vi "rcpacini_v_representation.vi"(6 "Variant in":variant, 7 "Shift Pressed?":bool, 8 "error in (no error)":errorcluster, 10 "QD Combo Box Ref":refnum<vi>, 11 "QD Launch VI Ref":refnum<vi>) -> (0 "error out":errorcluster, 4 "Variant out":variant)   [LabVIEW 2019]
doc: "Change the selected numeric or string control/constant representation, radix and modifiers using the quick drop text formatted as : \n<b>TYPE[ MODS...]</b>\n<b>TYPE</b> = 'u8', 'u16', 'u32', 'u64', 'i8', 'i16', 'i32', 'i64', 'sgl', 'dbl', 'ext'\n<b>MODS</b> = 'x':hex, 'd':dec/default, 'b':bin/backslash, 'h':hide inc/dec buttons \n\n<b>Examples:</b>\nNumeric selected + <b>\"u8 h x\"</b> = Unsigned 8-bit representation, display radix as hex and inc/dec buttons hidden\nString selected + <b>\"b\"</b> = Show display radix in backslash\n\nDefault Shortcut - [V]"
uses:
  <vilib>/numeric/LVNumericRepresentation.ctl
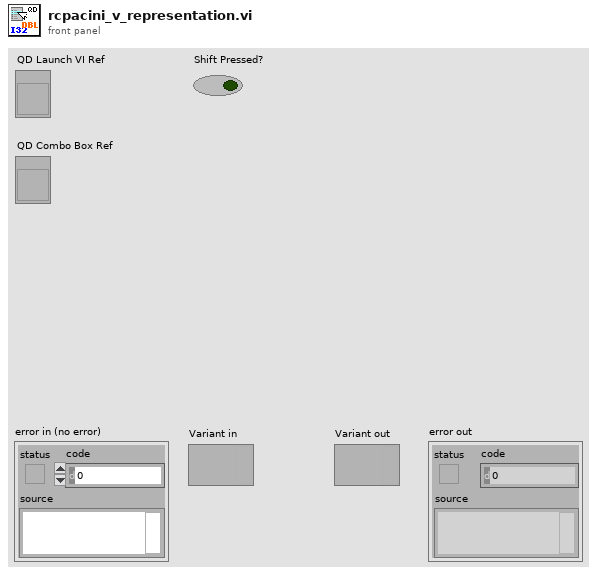
[diagram p1: front panel]
types:
  T1 = typedef "LVNumericRepresentation.ctl" = enum32{"Extended Precision", "Double Precision", "Single Precision", "Long", "Word", "Byte", "Unsigned Long", "Unsigned Word", "Unsigned Byte", "Complex Extended", "Complex Double", "Complex Single", "Quad", "Unsigned Quad", "Fixed-Point"}
  T2 = enum8{"none", "toggle", "decimal", "hex", "binary"}
  T3 = cluster{"DigitalCst":refnum<vi>[], "EnumCst":refnum<vi>[], "RingCst":refnum<vi>[], "StringCst":refnum<vi>[], "Digitals":refnum<vi>[], "Enums":refnum<vi>[], "Rings":refnum<vi>[], "Strings":refnum<vi>[]}
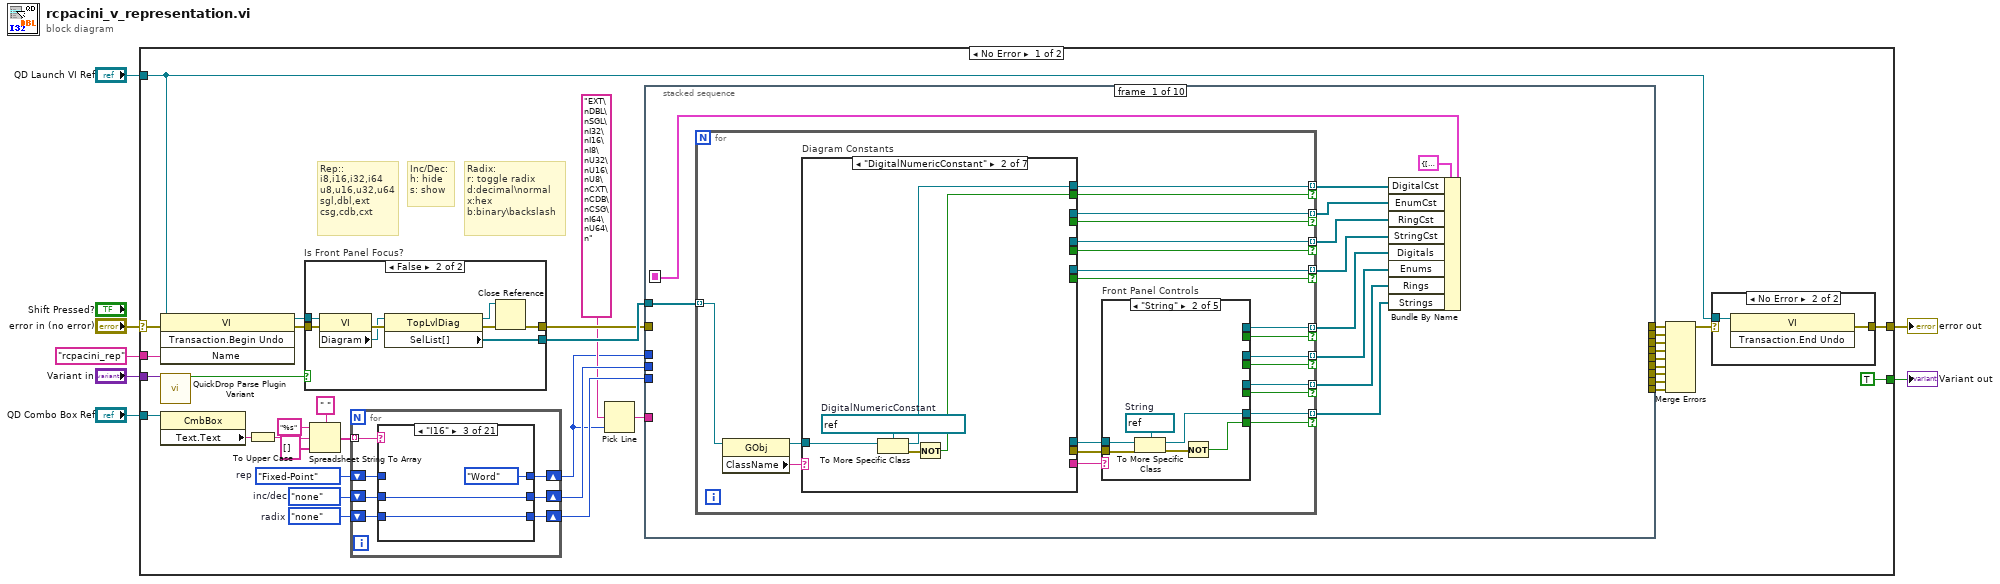
[diagram p0: block diagram]
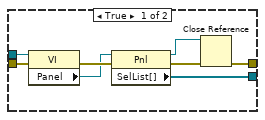
[diagram p2: hidden frame]
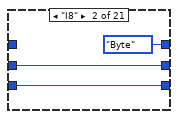
[diagram p4: hidden frame]
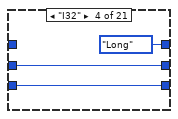
[diagram p5: hidden frame]
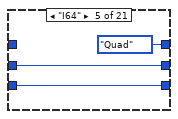
[diagram p6: hidden frame]
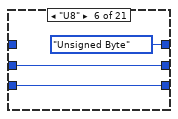
[diagram p7: hidden frame]
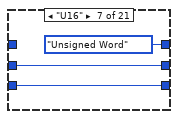
[diagram p8: hidden frame]
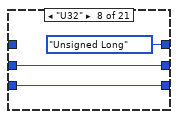
[diagram p9: hidden frame]
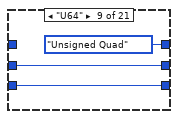
[diagram p10: hidden frame]
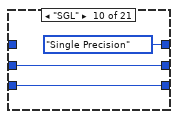
[diagram p11: hidden frame]
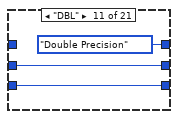
[diagram p12: hidden frame]
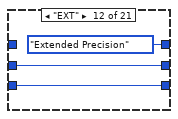
[diagram p13: hidden frame]
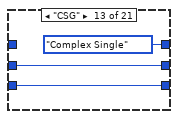
[diagram p14: hidden frame]
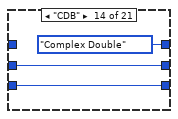
[diagram p15: hidden frame]
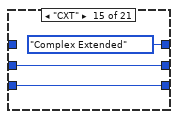
[diagram p16: hidden frame]
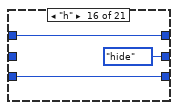
[diagram p17: hidden frame]
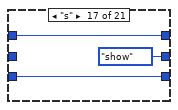
[diagram p18: hidden frame]
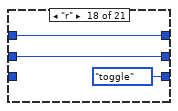
[diagram p19: hidden frame]
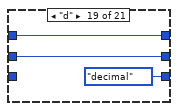
[diagram p20: hidden frame]
diagram:
  n1 = case shown="No Error" "error in (no error)" {
    selector: "error in (no error)" -> [w43 w621]
    tunnel: [w42 w621] -> w1
    tunnel: "QD Launch VI Ref" -> [w36 _]
    tunnel: "rcpacini_rep" ("Undo Name") -> [w41 _]
    tunnel: "Variant in" -> [w9 _]
    tunnel: "QD Combo Box Ref" -> [w37 _]
    tunnel: [TRUE _] -> w2
    frame No Error {
      w26 = enum8{"none", "show", "hide"}."none"  # inc/dec
      w27 = T2."none"  # radix
      w28 = LVNumericRepresentation."Fixed-Point"  # rep
      # "Radix:\nr: toggle radix\nd:decimal\\normal\nx:hex\nb:binary\\backslash"
      # "Inc/Dec:\nh: hide\ns: show"
      # "Rep::\ni8,i16,i32,i64\nu8,u16,u32,u64\nsgl,dbl,ext\ncsg,cdb,cxt"
      n2 = invoke class="VI" method="Transaction.Begin Undo"(reference=w36, error in=w43, "Name"=w41) -> (reference out=w39:refnum<vi>, error out=w40:errorcluster)  [unwired: 1 in, 2 out]
      n3 = call <vilib>:"QuickDrop Parse Plugin Variant.vi"("QDKS Variant in"=w9) -> ("QD Launch VI Panel?"=w8:bool)  [unwired: 12 in, 2 out]
      n4 = property class="CmbBox"(reference=w37) -> ("Text.Text"=w35:string)  [unwired: 1 in, 2 out]
      n5 = To Upper Case(1:w35) -> (0:w34:string)
      n6 = case "Is Front Panel Focus?" shown="False" w8 {
        tunnel: w40 -> [w51 w59]
        tunnel: w39 -> [w50 w58]
        tunnel: [w45 w53] -> w25
        tunnel: [w44 w52] -> w30
        frame True {
          n7 = property class="VI"(reference=w50, error in=w51) -> (error out=w49:errorcluster, "Panel"=w48:refnum<vi>)  [unwired: 1 out]
          n8 = property class="Pnl"(reference=w48, error in=w49) -> (reference out=w46:refnum<vi>, error out=w47:errorcluster, "SelList[]"=w44:refnum<vi>[])
          n9 = Close Reference(reference=w46, error in (no error)=w47) -> (error out=w45:errorcluster)
        }
        frame False {
          n10 = property class="VI"(reference=w58, error in=w59) -> (error out=w57:errorcluster, "Diagram"=w56:refnum<vi>)  [unwired: 1 out]
          n11 = property class="TopLvlDiag"(reference=w56, error in=w57) -> (reference out=w54:refnum<vi>, error out=w55:errorcluster, "SelList[]"=w52:refnum<vi>[])
          n12 = Close Reference(reference=w54, error in (no error)=w55) -> (error out=w53:errorcluster)
        }
      }
      n13 = Spreadsheet String To Array(delimiter (Tab)=" ", format string="%s", spreadsheet string=w34, array type (2D Dbl)=string[] []) -> (array=w29:string[])
      n14 = for {
        tunnel: w29 -> [w66] mode=indexing
        shift-right: [w64] -> w11
        shift-left: w28 -> [w65]
        shift-right: [w63] -> w23
        shift-left: w26 -> [w62]
        shift-right: [w60] -> w22
        shift-left: w27 -> [w61]
        n15 = case shown="\"I16\"" w66 {
          tunnel: w65 -> [w69 _ _ _ _ _ _ _ _ _ _ _ _ _ _ w114 w117 w120 w123 w126 w129]
          tunnel: [w69 LVNumericRepresentation."Byte" ("Representation") LVNumericRepresentation."Word" ("Representation") LVNumericRepresentation."Long" ("Representation") LVNumericRepresentation."Quad" ("Representation") LVNumericRepresentation."Unsigned Byte" ("Representation") LVNumericRepresentation."Unsigned Word" ("Representation") LVNumericRepresentation."Unsigned Long" ("Representation") LVNumericRepresentation."Unsigned Quad" ("Representation") LVNumericRepresentation."Single Precision" ("Representation") LVNumericRepresentation."Double Precision" ("Representation") LVNumericRepresentation."Extended Precision" ("Representation") LVNumericRepresentation."Complex Single" ("Representation") LVNumericRepresentation."Complex Double" ("Representation") LVNumericRepresentation."Complex Extended" ("Representation") w114 w117 w120 w123 w126 w129] -> w64
          tunnel: [w68 w71 w74 w77 w80 w83 w86 w89 w92 w95 w98 w101 w104 w107 w110 enum8{"none", "show", "hide"}."hide" ("inc/dec") enum8{"none", "show", "hide"}."show" ("inc/dec") w119 w122 w125 w128] -> w63
          tunnel: w62 -> [w68 w71 w74 w77 w80 w83 w86 w89 w92 w95 w98 w101 w104 w107 w110 _ _ w119 w122 w125 w128]
          tunnel: [w67 w70 w73 w76 w79 w82 w85 w88 w91 w94 w97 w100 w103 w106 w109 w113 w116 T2."toggle" ("radix") T2."decimal" ("radix") T2."hex" ("radix") T2."binary" ("radix")] -> w60
          tunnel: w61 -> [w67 w70 w73 w76 w79 w82 w85 w88 w91 w94 w97 w100 w103 w106 w109 w113 w116 _ _ _ _]
          frame Default {
          }
          frame "I8" {
          }
          frame "I16" {
          }
          frame "I32" {
          }
          frame "I64" {
          }
          frame "U8" {
          }
          frame "U16" {
          }
          frame "U32" {
          }
          frame "U64" {
          }
          frame "SGL" {
          }
          frame "DBL" {
          }
          frame "EXT" {
          }
          frame "CSG" {
          }
          frame "CDB" {
          }
          frame "CXT" {
          }
          frame "h" {
          }
          frame "s" {
          }
          frame "r" {
          }
          frame "d" {
          }
          frame "x" {
          }
          frame "b" {
          }
        }
      }
      n16 = Pick Line(multi-line string="EXT\nDBL\nSGL\nI32\nI16\nI8\nU32\nU16\nU8\nCXT\nCDB\nCSG\nI64\nU64\n", line index=w11) -> (output string=w10:string)  [unwired: 1 in]
      n17 = stacked-sequence {
        seq-local: [w130 _ _ _ _ _ _ _ _ _] -> [_ w220 w304 w334 w364 w414 w501 w532 w566 _]
        tunnel: w30 -> [w140 _ _ _ _ _ _ _ _ w616]
        tunnel: w25 -> [_ w219 w303 w333 w363 w413 w500 w531 w565 w615]
        tunnel: w11 -> [_ w224 w306 w336 _ w417 w503 w534 _ _]
        tunnel: w23 -> [_ w223 _ _ w365 w416 w502 w533 w567 _]
        tunnel: w22 -> [_ w222 _ _ w366 w415 _ _ w568 _]
        tunnel: [_ w218 _ _ _ _ _ _ _ _] -> w24
        tunnel: w10 -> [_ w221 w305 w335 _ _ _ _ _ _]
        tunnel: [_ _ w302 _ _ _ _ _ _ _] -> w21
        tunnel: [_ _ _ w332 _ _ _ _ _ _] -> w20
        tunnel: [_ _ _ _ w362 _ _ _ _ _] -> w19
        tunnel: [_ _ _ _ _ w412 _ _ _ _] -> w18
        tunnel: [_ _ _ _ _ _ w499 _ _ _] -> w17
        tunnel: [_ _ _ _ _ _ _ w530 _ _] -> w16
        tunnel: [_ _ _ _ _ _ _ _ w564 _] -> w15
        tunnel: [_ _ _ _ _ _ _ _ _ w614] -> w14
        frame #0 {
          n18 = for {
            tunnel: w140 -> [w162] mode=indexing
            tunnel: [w159] -> w139 mode=indexing if=w158
            tunnel: [w157] -> w138 mode=indexing if=w156
            tunnel: [w155] -> w137 mode=indexing if=w154
            tunnel: [w153] -> w136 mode=indexing if=w152
            tunnel: [w148] -> w132 mode=indexing if=w147
            tunnel: [w146] -> w135 mode=indexing if=w145
            tunnel: [w144] -> w134 mode=indexing if=w143
            tunnel: [w142] -> w133 mode=indexing if=w141
            n19 = property class="GObj"(reference=w162) -> (reference out=w160:refnum<vi>, "ClassName"=w161:string)  [unwired: 1 in, 1 out]
            n20 = case "Diagram Constants" shown="\"DigitalNumericConstant\"" w161 {
              selector: w161 -> [_ _ _ _ _ _ w216]
              tunnel: w160 -> [_ w190 w195 w200 w205 w214 w217]
              tunnel: [_ w189 _ _ _ _ _] -> w159
              tunnel: [_ w187 _ _ _ _ _] -> w158
              tunnel: [_ _ w193 _ _ _ _] -> w157
              tunnel: [_ _ w192 _ _ _ _] -> w156
              tunnel: [_ _ _ w198 _ _ _] -> w155
              tunnel: [_ _ _ w197 _ _ _] -> w154
              tunnel: [_ _ _ _ w203 _ _] -> w153
              tunnel: [_ _ _ _ w202 _ _] -> w152
              tunnel: [_ _ _ _ _ w209 w216] -> w149
              tunnel: [_ _ _ _ _ w208 w217] -> w151
              tunnel: [_ _ _ _ _ w207 _] -> w150
              frame Default {
              }
              frame "DigitalNumericConstant" {
                w191 = refnum<vi> refnum  # DigitalNumericConstant
                n21 = To More Specific Class(target class=w191, reference=w190) -> (specific class reference=w189:refnum<vi>, error out=w188:errorcluster)  [unwired: 1 in]
                n22 = Not(x=w188) -> (.not. x?=w187:bool)
              }
              frame "EnumConstant" {
                w196 = refnum<vi> refnum  # EnumConstant
                n23 = To More Specific Class(target class=w196, reference=w195) -> (specific class reference=w193:refnum<vi>, error out=w194:errorcluster)  [unwired: 1 in]
                n24 = Not(x=w194) -> (.not. x?=w192:bool)
              }
              frame "RingConstant" {
                w201 = refnum<vi> refnum  # RingConstant
                n25 = To More Specific Class(target class=w201, reference=w200) -> (specific class reference=w198:refnum<vi>, error out=w199:errorcluster)  [unwired: 1 in]
                n26 = Not(x=w199) -> (.not. x?=w197:bool)
              }
              frame "StringConstant" {
                w206 = refnum<vi> refnum  # StringConstant
                n27 = To More Specific Class(target class=w206, reference=w205) -> (specific class reference=w203:refnum<vi>, error out=w204:errorcluster)  [unwired: 1 in]
                n28 = Not(x=w204) -> (.not. x?=w202:bool)
              }
              frame "ControlTerminal" {
                w215 = refnum<vi> refnum  # ControlTerminal
                n29 = To More Specific Class(target class=w215, reference=w214) -> (specific class reference=w211:refnum<vi>, error out=w213:errorcluster)  [unwired: 1 in]
                n30 = property class="CtrlTerm"(reference=w211, error in=w213) -> (error out=w212:errorcluster, "Control"=w210:refnum<vi>)  [unwired: 1 out]
                n31 = property class="Ctl"(reference=w210, error in=w212) -> (reference out=w208:refnum<vi>, error out=w207:errorcluster, "ClassName"=w209:string)
              }
              frame "Digital", "Enum", "Ring", "String" {
              }
            }
            n32 = case "Front Panel Controls" shown="\"String\"" w149 {
              tunnel: w151 -> [_ w167 w173 w179 w185]
              tunnel: w150 -> [_ w166 w172 w178 w184]
              tunnel: [_ w164 _ _ _] -> w148
              tunnel: [_ w163 _ _ _] -> w147
              tunnel: [_ _ w170 _ _] -> w146
              tunnel: [_ _ w169 _ _] -> w145
              tunnel: [_ _ _ w176 _] -> w144
              tunnel: [_ _ _ w175 _] -> w143
              tunnel: [_ _ _ _ w182] -> w142
              tunnel: [_ _ _ _ w181] -> w141
              frame Default {
              }
              frame "String" {
                w168 = refnum<vi> refnum  # String
                n33 = To More Specific Class(target class=w168, reference=w167, error in=w166) -> (specific class reference=w164:refnum<vi>, error out=w165:errorcluster)
                n34 = Not(x=w165) -> (.not. x?=w163:bool)
              }
              frame "Digital" {
                w174 = refnum<vi> refnum  # Digital
                n35 = To More Specific Class(target class=w174, reference=w173, error in=w172) -> (specific class reference=w170:refnum<vi>, error out=w171:errorcluster)
                n36 = Not(x=w171) -> (.not. x?=w169:bool)
              }
              frame "Enum" {
                w180 = refnum<vi> refnum  # Enum
                n37 = To More Specific Class(target class=w180, reference=w179, error in=w178) -> (specific class reference=w176:refnum<vi>, error out=w177:errorcluster)
                n38 = Not(x=w177) -> (.not. x?=w175:bool)
              }
              frame "Ring" {
                w186 = refnum<vi> refnum  # Ring
                n39 = To More Specific Class(target class=w186, reference=w185, error in=w184) -> (specific class reference=w182:refnum<vi>, error out=w183:errorcluster)
                n40 = Not(x=w183) -> (.not. x?=w181:bool)
              }
            }
          }
          n41 = Bundle By Name(cluster=T3 {"DigitalCst"=[], "EnumCst"=[], "RingCst"=[], "StringCst"=[], "Digitals"=[], "Enums"=[], "Rings"=[], "Strings"=[]} ("refnums"), "DigitalCst"=w139, "EnumCst"=w138, "RingCst"=w137, "StringCst"=w136, "Digitals"=w135, "Enums"=w134, "Rings"=w133, "Strings"=w132) -> (w130:T3)
        }
        frame #1 {
          n42 = Unbundle By Name(w220) -> ("DigitalCst"=w225:refnum<vi>[])
          n43 = for {
            tunnel: w225 -> [w237] mode=indexing
            tunnel: w224 -> [w235]
            tunnel: w223 -> [_]
            tunnel: w222 -> [w234]
            tunnel: w219 -> [w236]
            tunnel: w221 -> [w230]
            shift-right: [w227] -> w218
            shift-left: w219 -> [w226]
            n44 = case shown="Default" w235 {
              selector: w235 -> [_ w298]
              tunnel: w237 -> [w295 w301]
              tunnel: w236 -> [w296 w300]
              tunnel: [w296 w299] -> w229
              tunnel: [w295 w297] -> w228
              frame "Fixed-Point" {
              }
              frame Default {
                n45 = property class="DigCnst"(reference=w301, error in=w300, "Representation"=w298) -> (reference out=w297:refnum<vi>, error out=w299:errorcluster)
              }
            }
            n46 = case shown="\"binary\"" w234 {
              tunnel: w229 -> [w247 w253 w264 w278 w294]
              tunnel: w228 -> [w246 w251 w262 w276 w293]
              tunnel: [w247 w255 w266 w280 w289] -> w233
              tunnel: [w246 w254 w265 w279 w287] -> w231
              frame "none" {
              }
              frame "decimal" {
                n47 = property class="DigCnst"(reference=w251, error in=w253) -> (reference out=w250:refnum<vi>, error out=w252:errorcluster, "Representation"=w249:T1)
                n48 = case shown="\"Long\"..\"Unsigned Byte\", \"Quad\", \"Unsigned Quad\"" w249 {
                  tunnel: [_ "%d" "%#_13g"] -> w248
                  frame "Fixed-Point" {
                  }
                  frame "Long".."Unsigned Byte", "Quad", "Unsigned Quad" {
                  }
                  frame "Extended Precision".."Single Precision", "Complex Extended".."Complex Single" {
                  }
                }
                n49 = property class="DigCnst"(reference=w250, error in=w252, "RadixVis"=TRUE ("Radix Visible?"), "FormatString"=w248) -> (reference out=w254:refnum<vi>, error out=w255:errorcluster)
              }
              frame "hex" {
                n50 = property class="DigCnst"(reference=w262, error in=w264) -> (reference out=w261:refnum<vi>, error out=w263:errorcluster, "Representation"=w260:T1)
                n51 = case shown="\"Extended Precision\"..\"Single Precision\", \"Complex Extended\"..\"Complex Single\"" w260 {
                  tunnel: [_ "%02x" "%04x" "%08x" "%016x" "%#_13g"] -> w259
                  frame "Fixed-Point" {
                  }
                  frame "Byte", "Unsigned Byte" {
                  }
                  frame "Word", "Unsigned Word" {
                  }
                  frame "Long", "Unsigned Long" {
                  }
                  frame "Quad", "Unsigned Quad" {
                  }
                  frame "Extended Precision".."Single Precision", "Complex Extended".."Complex Single" {
                  }
                }
                n52 = property class="DigCnst"(reference=w261, error in=w263, "RadixVis"=TRUE ("Radix Visible?"), "FormatString"=w259) -> (reference out=w265:refnum<vi>, error out=w266:errorcluster)
              }
              frame "binary" {
                n53 = property class="DigCnst"(reference=w276, error in=w278) -> (reference out=w275:refnum<vi>, error out=w277:errorcluster, "Representation"=w273:T1)
                n54 = case shown="\"Byte\", \"Unsigned Byte\"" w273 {
                  tunnel: [_ "%08b" "%016b" "%032b" "%064b" "%#_13g"] -> w274
                  frame "Fixed-Point" {
                  }
                  frame "Byte", "Unsigned Byte" {
                  }
                  frame "Word", "Unsigned Word" {
                  }
                  frame "Long", "Unsigned Long" {
                  }
                  frame "Quad", "Unsigned Quad" {
                  }
                  frame "Extended Precision".."Single Precision", "Complex Extended".."Complex Single" {
                  }
                }
                n55 = property class="DigCnst"(reference=w275, error in=w277, "RadixVis"=TRUE ("Radix Visible?"), "FormatString"=w274) -> (reference out=w279:refnum<vi>, error out=w280:errorcluster)
              }
              frame "toggle" {
                n56 = property class="DigCnst"(reference=w293, error in=w294) -> (reference out=w291:refnum<vi>, error out=w292:errorcluster, "RadixVis"=w290:bool)
                n57 = Not(x=w290) -> (.not. x?=w288:bool)
                n58 = property class="DigCnst"(reference=w291, error in=w292, "RadixVis"=w288) -> (reference out=w287:refnum<vi>, error out=w289:errorcluster)
              }
            }
            n59 = case shown="Default" w230 {
              selector: w230 -> [_ w239]
              tunnel: w233 -> [w238 w245]
              tunnel: [w238 w244] -> w232
              tunnel: w231 -> [_ w242]
              frame "" {
              }
              frame Default {
                n60 = property class="DigCnst"(reference=w242, error in=w245, "Label.Visible"=TRUE, "Label.Text"=w239) -> (reference out=w241:refnum<vi>, error out=w243:errorcluster)
                n61 = call "rcpacini_move_constant_label.vi"("error in (no error)"=w243, "Constant in"=w241) -> ("error out"=w244:errorcluster)  [unwired: 8 in, 1 out]
              }
            }
            n62 = Merge Errors(w226, w232) -> (w227:errorcluster)
          }
        }
        frame #2 {
          n63 = Unbundle By Name(w304) -> ("EnumCst"=w307:refnum<vi>[])
          n64 = for {
            tunnel: w307 -> [w316] mode=indexing
            tunnel: w306 -> [w314]
            tunnel: w303 -> [w315]
            tunnel: w305 -> [w311]
            shift-right: [w309] -> w302
            shift-left: w303 -> [w308]
            n65 = case shown="\"Unsigned Long\"..\"Unsigned Byte\"" w314 {
              selector: w314 -> [_ w328]
              tunnel: w316 -> [w325 w331]
              tunnel: w315 -> [w326 w330]
              tunnel: [w326 w329] -> w313
              tunnel: [w325 w327] -> w312
              frame Default {
              }
              frame "Unsigned Long".."Unsigned Byte" {
                n66 = property class="EnmCnst"(reference=w331, error in=w330, "Representation"=w328) -> (reference out=w327:refnum<vi>, error out=w329:errorcluster)
              }
            }
            n67 = case shown="Default" w311 {
              selector: w311 -> [_ w318]
              tunnel: w313 -> [w317 w324]
              tunnel: [w317 w323] -> w310
              tunnel: w312 -> [_ w321]
              frame "" {
              }
              frame Default {
                n68 = property class="EnmCnst"(reference=w321, error in=w324, "Label.Visible"=TRUE, "Label.Text"=w318) -> (reference out=w320:refnum<vi>, error out=w322:errorcluster)
                n69 = call "rcpacini_move_constant_label.vi"("error in (no error)"=w322, "Constant in"=w320) -> ("error out"=w323:errorcluster)  [unwired: 8 in, 1 out]
              }
            }
            n70 = Merge Errors(w308, w310) -> (w309:errorcluster)
          }
        }
        frame #3 {
          n71 = Unbundle By Name(w334) -> ("RingCst"=w337:refnum<vi>[])
          n72 = for {
            tunnel: w337 -> [w346] mode=indexing
            tunnel: w336 -> [w344]
            tunnel: w333 -> [w345]
            tunnel: w335 -> [w342]
            shift-right: [w339] -> w332
            shift-left: w333 -> [w338]
            n73 = case shown="Default" w344 {
              selector: w344 -> [_ w358]
              tunnel: w346 -> [w355 w361]
              tunnel: w345 -> [w356 w360]
              tunnel: [w356 w359] -> w343
              tunnel: [w355 w357] -> w340
              frame "Complex Extended".."Complex Single", "Fixed-Point" {
              }
              frame Default {
                n74 = property class="RngCnst"(reference=w361, error in=w360, "Representation"=w358) -> (reference out=w357:refnum<vi>, error out=w359:errorcluster)
              }
            }
            n75 = case shown="Default" w342 {
              selector: w342 -> [_ w348]
              tunnel: w343 -> [w347 w354]
              tunnel: [w347 w353] -> w341
              tunnel: w340 -> [_ w351]
              frame "" {
              }
              frame Default {
                n76 = property class="RngCnst"(reference=w351, error in=w354, "Label.Visible"=TRUE, "Label.Text"=w348) -> (reference out=w350:refnum<vi>, error out=w352:errorcluster)
                n77 = call "rcpacini_move_constant_label.vi"("error in (no error)"=w352, "Constant in"=w350) -> ("error out"=w353:errorcluster)  [unwired: 8 in, 1 out]
              }
            }
            n78 = Merge Errors(w338, w341) -> (w339:errorcluster)
          }
        }
        frame #4 {
          n79 = Unbundle By Name(w364) -> ("StringCst"=w367:refnum<vi>[])
          n80 = for {
            tunnel: w367 -> [w372] mode=indexing
            tunnel: w366 -> [w375]
            tunnel: w363 -> [w374]
            tunnel: w365 -> [w370]
            shift-right: [w369] -> w362
            shift-left: w363 -> [w368]
            n81 = case shown="\"hide\"" w370 {
              tunnel: w374 -> [w377 w383 w388]
              tunnel: [w377 w382 w387] -> w373
              tunnel: w372 -> [w378 w381 w386]
              tunnel: [w378 w380 w385] -> w371
              frame "none" {
              }
              frame "show" {
                n82 = property class="StrCnst"(reference=w381, error in=w383, "ScrollVis"=TRUE ("Scrollbar Visible?")) -> (reference out=w380:refnum<vi>, error out=w382:errorcluster)
              }
              frame "hide" {
                n83 = property class="StrCnst"(reference=w386, error in=w388, "ScrollVis"=FALSE ("Scrollbar Visible?")) -> (reference out=w385:refnum<vi>, error out=w387:errorcluster)
              }
            }
            n84 = case shown="\"toggle\"" w375 {
              tunnel: w371 -> [_ w396 w399 w404 w409]
              tunnel: w373 -> [w389 w395 w400 w405 w410]
              tunnel: [w389 w390 w401 w406 w411] -> w376
              frame "none" {
              }
              frame "toggle" {
                n85 = property class="StrCnst"(reference=w396, error in=w395) -> (reference out=w393:refnum<vi>, error out=w394:errorcluster, "DisplayFormatVisibility"=w392:bool)
                n86 = Not(x=w392) -> (.not. x?=w391:bool)
                n87 = property class="StrCnst"(reference=w393, error in=w394, "DisplayFormatVisibility"=w391) -> (error out=w390:errorcluster)  [unwired: 1 out]
              }
              frame "decimal" {
                w397 = u32 0  # normal
                n88 = property class="StrCnst"(reference=w399, error in=w400, "DisplayFormatVisibility"=TRUE ("Display Format Visible?"), "DispStyle"=w397) -> (error out=w401:errorcluster)  [unwired: 1 out]
              }
              frame "hex" {
                w402 = u32 3  # hex
                n89 = property class="StrCnst"(reference=w404, error in=w405, "DisplayFormatVisibility"=TRUE ("Display Format Visible?"), "DispStyle"=w402) -> (error out=w406:errorcluster)  [unwired: 1 out]
              }
              frame "binary" {
                w407 = u32 1  # backslash
                n90 = property class="StrCnst"(reference=w409, error in=w410, "DisplayFormatVisibility"=TRUE ("Display Format Visible?"), "DispStyle"=w407) -> (error out=w411:errorcluster)  [unwired: 1 out]
              }
            }
            n91 = Merge Errors(w368, w376) -> (w369:errorcluster)
          }
        }
        frame #5 {
          n92 = Unbundle By Name(w414) -> ("Digitals"=w418:refnum<vi>[])
          n93 = for {
            tunnel: w418 -> [w430] mode=indexing
            tunnel: w417 -> [w428]
            tunnel: w416 -> [w425]
            tunnel: w415 -> [w422]
            tunnel: w413 -> [w429]
            shift-right: [w420] -> w412
            shift-left: w413 -> [w419]
            n94 = case shown="Default" w428 {
              selector: w428 -> [_ w495]
              tunnel: w430 -> [w492 w498]
              tunnel: w429 -> [w493 w497]
              tunnel: [w493 w496] -> w427
              tunnel: [w492 w494] -> w426
              frame "Fixed-Point" {
              }
              frame Default {
                n95 = property class="DigNum"(reference=w498, error in=w497, "Rep"=w495) -> (reference out=w494:refnum<vi>, error out=w496:errorcluster)
              }
            }
            n96 = case shown="\"hide\"" w425 {
              tunnel: w427 -> [w481 w486 w491]
              tunnel: w426 -> [w480 w485 w490]
              tunnel: [w481 w483 w488] -> w424
              tunnel: [w480 w482 w487] -> w423
              frame "none" {
              }
              frame "show" {
                n97 = property class="DigNum"(reference=w485, error in=w486, "IncDecVis"=TRUE ("Increment/Decrement Visible?")) -> (reference out=w482:refnum<vi>, error out=w483:errorcluster)
              }
              frame "hide" {
                n98 = property class="DigNum"(reference=w490, error in=w491, "IncDecVis"=FALSE ("Increment/Decrement Visible?")) -> (reference out=w487:refnum<vi>, error out=w488:errorcluster)
              }
            }
            n99 = case shown="\"binary\"" w422 {
              tunnel: w424 -> [w432 w438 w449 w463 w479]
              tunnel: w423 -> [w431 w436 w447 w461 w478]
              tunnel: [w432 w440 w451 w465 w474] -> w421
              tunnel: [w431 w439 w450 w464 w472] -> _
              frame "none" {
              }
              frame "decimal" {
                n100 = property class="DigNum"(reference=w436, error in=w438) -> (reference out=w435:refnum<vi>, error out=w437:errorcluster, "Rep"=w434:T1)
                n101 = case shown="\"Long\"..\"Unsigned Byte\", \"Quad\", \"Unsigned Quad\"" w434 {
                  tunnel: [_ "%d" "%#_13g"] -> w433
                  frame "Fixed-Point" {
                  }
                  frame "Long".."Unsigned Byte", "Quad", "Unsigned Quad" {
                  }
                  frame "Extended Precision".."Single Precision", "Complex Extended".."Complex Single" {
                  }
                }
                n102 = property class="DigNum"(reference=w435, error in=w437, "RadixVis"=TRUE ("Radix Visible?"), "FormatString"=w433) -> (reference out=w439:refnum<vi>, error out=w440:errorcluster)
              }
              frame "hex" {
                n103 = property class="DigNum"(reference=w447, error in=w449) -> (reference out=w446:refnum<vi>, error out=w448:errorcluster, "Rep"=w445:T1)
                n104 = case shown="\"Extended Precision\"..\"Single Precision\", \"Complex Extended\"..\"Complex Single\"" w445 {
                  tunnel: [_ "%02x" "%04x" "%08x" "%016x" "%#_13g"] -> w444
                  frame "Fixed-Point" {
                  }
                  frame "Byte", "Unsigned Byte" {
                  }
                  frame "Word", "Unsigned Word" {
                  }
                  frame "Long", "Unsigned Long" {
                  }
                  frame "Quad", "Unsigned Quad" {
                  }
                  frame "Extended Precision".."Single Precision", "Complex Extended".."Complex Single" {
                  }
                }
                n105 = property class="DigNum"(reference=w446, error in=w448, "RadixVis"=TRUE ("Radix Visible?"), "FormatString"=w444) -> (reference out=w450:refnum<vi>, error out=w451:errorcluster)
              }
              frame "binary" {
                n106 = property class="DigNum"(reference=w461, error in=w463) -> (reference out=w460:refnum<vi>, error out=w462:errorcluster, "Rep"=w458:T1)
                n107 = case shown="\"Quad\", \"Unsigned Quad\"" w458 {
                  tunnel: [_ "%08b" "%016b" "%032b" "%064b" "%#_13g"] -> w459
                  frame "Fixed-Point" {
                  }
                  frame "Byte", "Unsigned Byte" {
                  }
                  frame "Word", "Unsigned Word" {
                  }
                  frame "Long", "Unsigned Long" {
                  }
                  frame "Quad", "Unsigned Quad" {
                  }
                  frame "Extended Precision".."Single Precision", "Complex Extended".."Complex Single" {
                  }
                }
                n108 = property class="DigNum"(reference=w460, error in=w462, "RadixVis"=TRUE ("Radix Visible?"), "FormatString"=w459) -> (reference out=w464:refnum<vi>, error out=w465:errorcluster)
              }
              frame "toggle" {
                n109 = property class="DigNum"(reference=w478, error in=w479) -> (reference out=w476:refnum<vi>, error out=w477:errorcluster, "RadixVis"=w475:bool)
                n110 = Not(x=w475) -> (.not. x?=w473:bool)
                n111 = property class="DigNum"(reference=w476, error in=w477, "RadixVis"=w473) -> (reference out=w472:refnum<vi>, error out=w474:errorcluster)
              }
            }
            n112 = Merge Errors(w419, w421) -> (w420:errorcluster)
          }
        }
        frame #6 {
          n113 = Unbundle By Name(w501) -> ("Enums"=w504:refnum<vi>[])
          n114 = for {
            tunnel: w504 -> [w513] mode=indexing
            tunnel: w503 -> [w511]
            tunnel: w500 -> [w512]
            tunnel: w502 -> [w507]
            shift-right: [w506] -> w499
            shift-left: w500 -> [w505]
            n115 = case shown="\"Unsigned Long\"..\"Unsigned Byte\"" w511 {
              selector: w511 -> [_ w526]
              tunnel: w513 -> [w523 w529]
              tunnel: w512 -> [w524 w528]
              tunnel: [w524 w527] -> w510
              tunnel: [w523 w525] -> w508
              frame Default {
              }
              frame "Unsigned Long".."Unsigned Byte" {
                n116 = property class="Enum"(reference=w529, error in=w528, "Rep"=w526) -> (reference out=w525:refnum<vi>, error out=w527:errorcluster)
              }
            }
            n117 = case shown="\"show\"" w507 {
              tunnel: w510 -> [w514 w518 w522]
              tunnel: w508 -> [_ w517 w521]
              tunnel: [w514 w515 w519] -> w509
              frame "none" {
              }
              frame "show" {
                n118 = property class="Enum"(reference=w517, error in=w518, "IncDecVis"=TRUE ("Increment/Decrement Visible?")) -> (error out=w515:errorcluster)  [unwired: 1 out]
              }
              frame "hide" {
                n119 = property class="Enum"(reference=w521, error in=w522, "IncDecVis"=FALSE ("Increment/Decrement Visible?")) -> (error out=w519:errorcluster)  [unwired: 1 out]
              }
            }
            n120 = Merge Errors(w505, w509) -> (w506:errorcluster)
          }
        }
        frame #7 {
          n121 = Unbundle By Name(w532) -> ("Rings"=w535:refnum<vi>[])
          n122 = for {
            tunnel: w535 -> [w544] mode=indexing
            tunnel: w534 -> [w542]
            tunnel: w531 -> [w543]
            tunnel: w533 -> [w538]
            shift-right: [w537] -> w530
            shift-left: w531 -> [w536]
            n123 = case shown="Default" w542 {
              selector: w542 -> [_ w560]
              tunnel: w544 -> [w557 w563]
              tunnel: w543 -> [w558 w562]
              tunnel: [w558 w561] -> w541
              tunnel: [w557 w559] -> w539
              frame "Complex Extended".."Complex Single", "Fixed-Point" {
              }
              frame Default {
                n124 = property class="Ring"(reference=w563, error in=w562, "Rep"=w560) -> (reference out=w559:refnum<vi>, error out=w561:errorcluster)
              }
            }
            n125 = case shown="\"show\"" w538 {
              tunnel: w541 -> [w546 w551 w556]
              tunnel: w539 -> [w545 w550 w555]
              tunnel: [w546 w548 w553] -> w540
              tunnel: [w545 w547 w552] -> _
              frame "none" {
              }
              frame "show" {
                n126 = property class="Ring"(reference=w550, error in=w551, "IncDecVis"=TRUE ("Increment/Decrement Visible?")) -> (reference out=w547:refnum<vi>, error out=w548:errorcluster)
              }
              frame "hide" {
                n127 = property class="Ring"(reference=w555, error in=w556, "IncDecVis"=FALSE ("Increment/Decrement Visible?")) -> (reference out=w552:refnum<vi>, error out=w553:errorcluster)
              }
            }
            n128 = Merge Errors(w536, w540) -> (w537:errorcluster)
          }
        }
        frame #8 {
          n129 = Unbundle By Name(w566) -> ("Strings"=w569:refnum<vi>[])
          n130 = for {
            tunnel: w569 -> [w575] mode=indexing
            tunnel: w568 -> [w577]
            tunnel: w565 -> [w576]
            tunnel: w567 -> [w572]
            shift-right: [w571] -> w564
            shift-left: w565 -> [w570]
            n131 = case shown="\"show\"" w572 {
              tunnel: w576 -> [w579 w585 w590]
              tunnel: [w579 w584 w589] -> w574
              tunnel: w575 -> [w580 w583 w588]
              tunnel: [w580 w582 w587] -> w573
              frame "none" {
              }
              frame "show" {
                n132 = property class="Str"(reference=w583, error in=w585, "VScrollVis"=TRUE ("Scrollbar Visible?")) -> (reference out=w582:refnum<vi>, error out=w584:errorcluster)
              }
              frame "hide" {
                n133 = property class="Str"(reference=w588, error in=w590, "VScrollVis"=FALSE ("Scrollbar Visible?")) -> (reference out=w587:refnum<vi>, error out=w589:errorcluster)
              }
            }
            n134 = case shown="\"hex\"" w577 {
              tunnel: w573 -> [_ w598 w601 w606 w611]
              tunnel: w574 -> [w591 w597 w602 w607 w612]
              tunnel: [w591 w592 w603 w608 w613] -> w578
              frame "none" {
              }
              frame "toggle" {
                n135 = property class="Str"(reference=w598, error in=w597) -> (reference out=w595:refnum<vi>, error out=w596:errorcluster, "DisplayFormatVisibility"=w594:bool)
                n136 = Not(x=w594) -> (.not. x?=w593:bool)
                n137 = property class="Str"(reference=w595, error in=w596, "DisplayFormatVisibility"=w593) -> (error out=w592:errorcluster)  [unwired: 1 out]
              }
              frame "decimal" {
                w599 = u32 0  # normal
                n138 = property class="Str"(reference=w601, error in=w602, "DisplayFormatVisibility"=TRUE ("Display Format Visible?"), "Display Style"=w599) -> (error out=w603:errorcluster)  [unwired: 1 out]
              }
              frame "hex" {
                w604 = u32 3  # hex
                n139 = property class="Str"(reference=w606, error in=w607, "DisplayFormatVisibility"=TRUE ("Display Format Visible?"), "Display Style"=w604) -> (error out=w608:errorcluster)  [unwired: 1 out]
              }
              frame "binary" {
                w609 = u32 1  # backslash
                n140 = property class="Str"(reference=w611, error in=w612, "DisplayFormatVisibility"=TRUE ("Display Format Visible?"), "Display Style"=w609) -> (error out=w613:errorcluster)  [unwired: 1 out]
              }
            }
            n141 = Merge Errors(w570, w578) -> (w571:errorcluster)
          }
        }
        frame #9 {
          n142 = Close Reference(reference=w616, error in (no error)=w615) -> (error out=w614:errorcluster)
        }
      }
      n143 = Merge Errors(w24, w21, w20, w19, w18, w17, w16, w15, w14) -> (w13:errorcluster)
      n144 = case shown="No Error" w13 {
        tunnel: w36 -> [w617 w619]
        tunnel: [w618 w620] -> w42
        frame Error {
          n145 = invoke class="VI" method="Transaction.Fail"(reference=w617) -> (error out=w618:errorcluster)  [unwired: 2 in, 2 out]
        }
        frame No Error {
          n146 = invoke class="VI" method="Transaction.End Undo"(reference=w619) -> (error out=w620:errorcluster)  [unwired: 2 in, 2 out]
        }
      }
    }
    frame Error {
    }
  }
  "error out" <- w1
  "Variant out" <- w2
